vi "Configure SMU Positive Over Voltage Remote Protection.vi"(8 "error in (no error)":errorcluster {"code" format="%.0x"}, 9 "Positive OVRP Level (0.0 volts)":dbl format="%^.3e", 10 "Channel Name (1)":string="1", 11 "VISA resource name":refnum<visa-resource-name>) -> (0 "error out":errorcluster {"code" format="%.0x"}, 3 "VISA resource name out":refnum<visa-resource-name>)   [LabVIEW 2010, in "Agilent N6700 Series.lvlib"]
doc: "Sets the positive over-voltage remote protection (OVP) level of the output channel. \n\n<b>Note:</b>\n\nThis VI only applies to models N678xA SMU."
uses:
  Agilent N6700 Series.lvlib
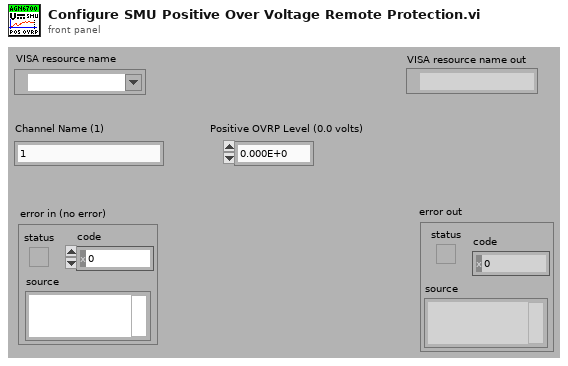
[diagram p1: front panel]
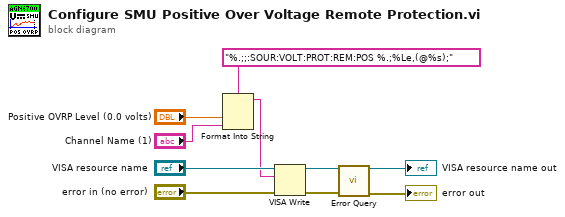
[diagram p0: block diagram]
diagram:
  n1 = Format Into String(format string="%.;;:SOUR:VOLT:PROT:REM:POS %.;%Le,(@%s);", "Positive OVRP Level (0.0 volts)", "Channel Name (1)") -> (resulting string=w4:string)  [unwired: 2 in, 1 out]
  n2 = VISA Write(VISA resource name="VISA resource name", write buffer=w4, error in (no error)="error in (no error)") -> (VISA resource name out=w6:refnum<visa-resource-name>, error out=w5:errorcluster)  [unwired: 1 out]
  n3 = call "Error Query.vi"("VISA resource name"=w6, "error in (no error)"=w5) -> ("VISA resource name out"=→"VISA resource name out":refnum<visa-resource-name>, "error out"=→"error out":errorcluster)  [unwired: 10 in, 2 out]
